vi "Read configuration.vi"(7 "force loading?":bool=TRUE, 8 "error in (no error)":errorcluster, 11 "Cascade in":refnum<class "Cascade.lvclass">) -> (0 "error out":errorcluster, 3 "Cascade out":refnum<class "Cascade.lvclass">)   [LabVIEW 2012, in "Cascade.lvclass"]
doc: "Reads the XML-based configuration file and populates the configuration cluster accordingly. Configuration file name is <component ID>.xml."
uses:
  Cascade.lvclass
  <vilib>/Distrio/Murmex/Murmex/Murmex.lvclass
  Cascade.lvclass/Cascade.ctl
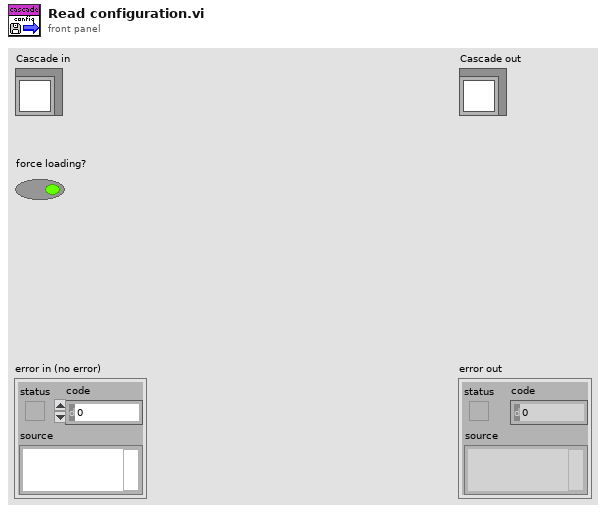
[diagram p1: front panel]
types:
  T1 = typedef "Cascade.lvclass/configuration.ctl" = cluster{"Numeric":dbl}
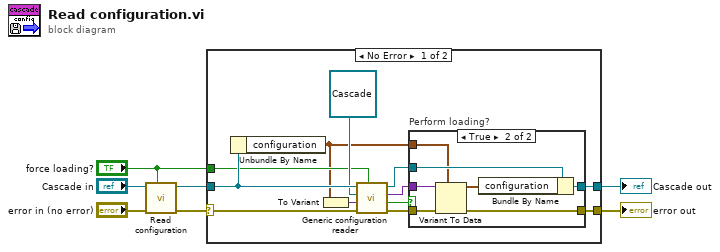
[diagram p0: block diagram]
diagram:
  n1 = call-parent "Read configuration.vi"("force loading?"="force loading?", "error in (no error)"="error in (no error)", "Murmex in"="Cascade in") -> ("error out"=w5:errorcluster, "Murmex out"=w3:refnum<class "Cascade.lvclass">)  [unwired: 7 in]
  n2 = case shown="No Error" w5 {
    selector: w5 -> [w18 w30]
    tunnel: [w16 w30] -> w4
    tunnel: w3 -> [w15 w29]
    tunnel: "force loading?" -> [w13 _]
    tunnel: [w9 w29] -> w1
    frame No Error {
      n3 = Unbundle By Name(w15) -> ("configuration"=w10:T1)
      n4 = To Variant(anything=w10) -> (Variant=w19:variant)
      n5 = call <vilib>:"Generic configuration reader.vi"("force loading?"=w13, "error in (no error)"=w18, "configuration cluster variant"=w19, "inheritance level"=refnum<class "Cascade.lvclass"> refnum ("Cascade.lvclass"), "Murmex in"=w15) -> ("error out"=w17:errorcluster, "loaded?"=w8:bool, "configuration data (variant)"=w11:variant, "Murmex out"=w12:refnum<class "Cascade.lvclass">)  [unwired: 3 in]
      n6 = case "Perform loading?" shown="True" w8 {
        tunnel: [w20 w26] -> w9
        tunnel: [w21 w28] -> w16
        tunnel: w17 -> [w21 w27]
        tunnel: w12 -> [w20 w25]
        tunnel: w11 -> [_ w24]
        tunnel: w10 -> [_ w23]
        frame False {
        }
        frame True {
          n7 = Variant To Data(error in=w27, type=w23, Variant=w24) -> (data=w22:T1, error out=w28:errorcluster)
          n8 = Bundle By Name(cluster=w25, "configuration"=w22) -> (w26:refnum<class "Cascade.lvclass">)
        }
      }
    }
    frame Error {
    }
  }
  "error out" <- w4
  "Cascade out" <- w1
